vi "PlotGraph.vi"(0 "reference in":refnum<class "HTMLPlot.lvclass">, 5 "error in (no error)":errorcluster) -> (14 "reference out":refnum<class "HTMLPlot.lvclass">, 19 "error out":errorcluster)   [LabVIEW 2019, in "HTMLPlot.lvclass"]
uses:
  HTMLPlot.lvclass
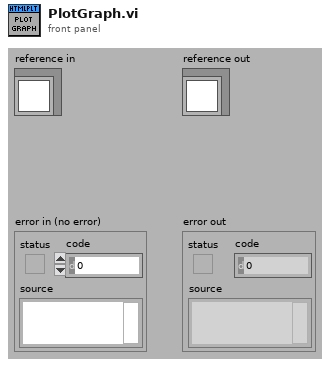
[diagram p1: front panel]
types:
  T1 = typedef "HTMLPlot.lvclass/ObjectAttributes.ctl" = cluster{"Attribute1":dbl, "GraphContainer":refnum<k7>, "ChartScriptFile":string, "UtilScriptFile(demoData)":string, "BaseHTML":string, "GenericProperties":cluster{"PlotType":T2, "PlotTitle":string, "XLabel":string, "YLabel":string, "ShowToolTip":bool}, "LegendProperties":cluster{"Show":bool, "Position":T3}, "BarPlot":cluster{"Dataset":dbl[][], "DatasetLabels":string[], "XLabels":string[], "PlotColours":u32[], "Stacked":bool}, "PiePlot":cluster{"Dataset":dbl[][], "DatasetLabels":string[], "PlotColours":u32[], "DoughnutStyle":bool, "PlotLabels":string[]}, "connection ID":refnum<k5>, "PortID":u64}
  T2 = typedef "HTMLPlot.lvclass/PlotType.ctl" = enum16{"bar", "line", "pie"}
  T3 = typedef "HTMLPlot.lvclass/LegendPosition.ctl" = enum16{"top", "right", "left", "bottom"}
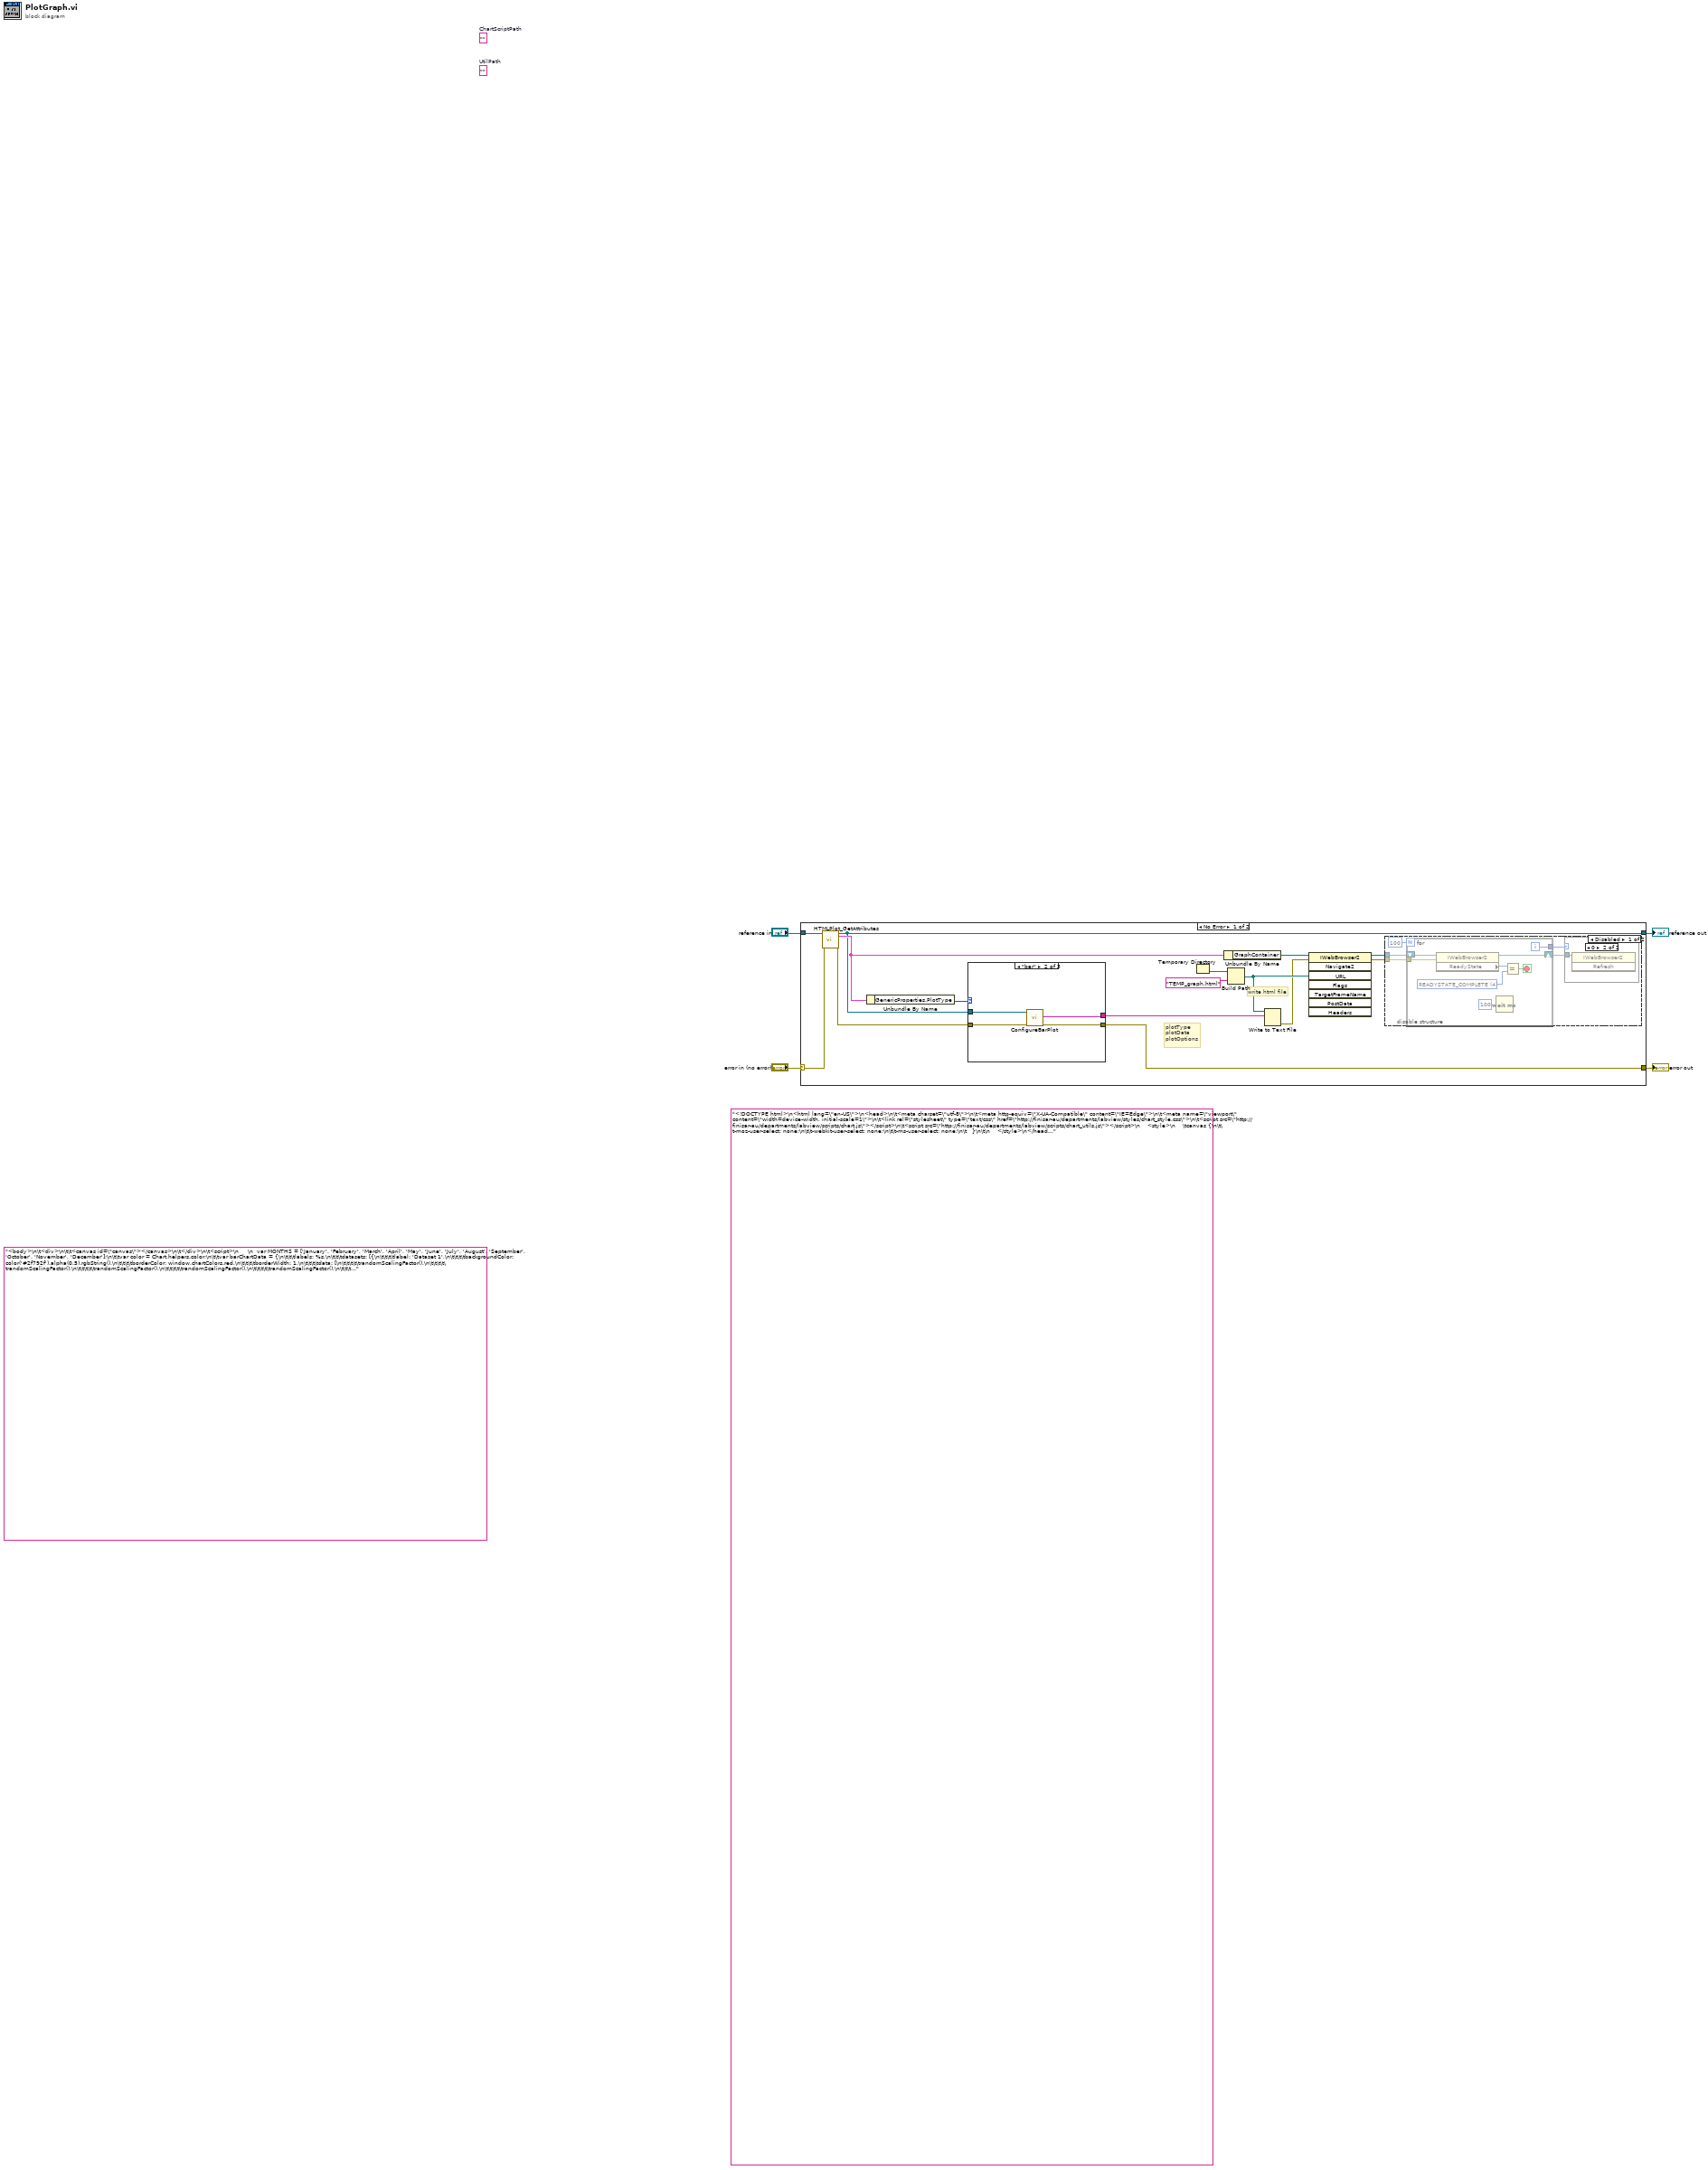
[diagram p0: block diagram]
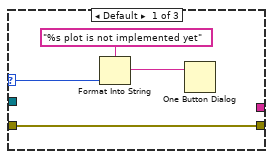
[diagram p2: hidden frame]
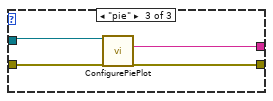
[diagram p3: hidden frame]
diagram:
  (unwired) ""  # UtilPath
  (unwired) ""  # ChartScriptPath
  (unwired) "<body>\n\t<div>\n\t\t<canvas id=\"canvas\"></canvas>\n\t</div>\n\t<script>\n     \n  var MONTHS = ['January', 'February', 'March', 'April', 'May', 'June', 'July', 'August', 'September', 'October', 'November', 'December'];\n\t\tvar color = Chart.helpers.color;\n\t\tvar barChartData = {\n\t\t\tlabels: %s,\n\t\t\tdatasets: [{\n\t\t\t\tlabel: 'Dataset 1',\n\t\t\t\tbackgroundColor: color('#2f792f').alpha(0.5).rgbString(),\n\t\t\t\tborderColor: window.chartColors.red,\n\t\t\t\tborderWidth: 1,\n\t\t\t\tdata: [\n\t\t\t\t\trandomScalingFactor(),\n\t\t\t\t\trandomScalingFactor(),\n\t\t\t\t\trandomScalingFactor(),\n\t\t\t\t\trandomScalingFactor(),\n\t\t\t\t\trandomScalingFactor(),\n\t\t\t\t\trandomScalingFactor(),\n\t\t\t\t\trandomScalingFactor()\n\t\t\t\t]\n\t\t\t}, {\n\t\t\t\tlabel: 'Dataset 2',\n\t\t\t\tbackgroundColor: color(window.chartColors.blue).alpha(0.5).rgbString(),\n\t\t\t\tborderColor: window.chartColors.blue,\n\t\t\t\tborderWidth: 1,\n\t\t\t\tdata: [\n\t\t\t\t\trandomScalingFactor(),\n\t\t\t\t\trandomScalingFactor(),\n\t\t\t\t\trandomScalingFactor(),\n\t\t\t\t\trandomScalingFactor(),\n\t\t\t\t\trandomScalingFactor(),\n\t\t\t\t\trandomScalingFactor(),\n\t\t\t\t\trandomScalingFactor()\n\t\t\t\t]\n\t\t\t}]\n\n\t\t};\n\n\t\twindow.onload = function() {\n\t\t\t//var ctx = document.getElementById('canvas').getContext('2d');\n\t\t\twindow.myBar = new Chart('canvas', {\n\t\t\t\ttype: 'bar',\n\t\t\t\tdata: barChartData,\n\t\t\t\toptions: {\n\t\t\t\t\tresponsive: true,\n\t\t\t\t\tlegend: {\n\t\t\t\t\t\tposition: 'top'\n\t\t\t\t\t},\n\t\t\t\t\ttitle: {\n\t\t\t\t\t\tdisplay: true,\n\t\t\t\t\t\ttext: 'Chart.js Bar Chart'\n\t\t\t\t\t},\n                    scales: {\n\t\t\t\t\t\txAxes: [{\n\t\t\t\t\t\t\tstacked: true,\n\t\t\t\t\t\t}],\n\t\t\t\t\t\tyAxes: [{\n\t\t\t\t\t\t\tstacked: true\n\t\t\t\t\t\t}]\n\t\t\t\t\t}\n\t\t\t\t}\n\t\t\t});\n\n\t\t};\n\n\n\t</script>\n</body>\n\n</html>\n\n\n"
  (unwired) "<!DOCTYPE html>\n<html lang=\"en-US\">\n<head>\n\t<meta charset=\"utf-8\">\n\t<meta http-equiv=\"X-UA-Compatible\" content=\"IE=Edge\">\n\t<meta name=\"viewport\" content=\"width=device-width, initial-scale=1\">\n\t<link rel=\"stylesheet\" type=\"text/css\" href=\"http://finisar-au/departments/labview/styles/chart_style.css\">\n\t<script src=\"http://finisar-au/departments/labview/scripts/chart.js\"></script>\n\t<script src=\"http://finisar-au/departments/labview/scripts/chart_utils.js\"></script>\n    <style>\n    \tcanvas {\n\t\t-moz-user-select: none;\n\t\t-webkit-user-select: none;\n\t\t-ms-user-select: none;\n\t   }\n\t\n    </style>\n</head>\n\n\n\n<body>\n\t<div id=\"container\" style=\"width: 75%;\">\n\t\t<canvas id=\"canvas\"></canvas>\n\t</div>\n\t<button id=\"randomizeData\">Randomize Data</button>\n\t<button id=\"addDataset\">Add Dataset</button>\n\t<button id=\"removeDataset\">Remove Dataset</button>\n\t<button id=\"addData\">Add Data</button>\n\t<button id=\"removeData\">Remove Data</button>\n\t<script>\n\t\tvar MONTHS = ['January', 'February', 'March', 'April', 'May', 'June', 'July', 'August', 'September', 'October', 'November', 'December'];\n\t\tvar color = Chart.helpers.color;\n        var Dataset1Color='#2f792f';\n\t\tvar barChartData = {\n\t\t\tlabels: ['January', 'February', 'March', 'April', 'May', 'June', 'July'],\n\t\t\tdatasets: [{\n\t\t\t\tlabel: 'Dataset 1',\n\t\t\t\tbackgroundColor: color('#2f792f').alpha(0.5).rgbString(),\n\t\t\t\tborderColor: window.chartColors.red,\n\t\t\t\tborderWidth: 1,\n\t\t\t\tdata: [\n\t\t\t\t\trandomScalingFactor(),\n\t\t\t\t\trandomScalingFactor(),\n\t\t\t\t\trandomScalingFactor(),\n\t\t\t\t\trandomScalingFactor(),\n\t\t\t\t\trandomScalingFactor(),\n\t\t\t\t\trandomScalingFactor(),\n\t\t\t\t\trandomScalingFactor()\n\t\t\t\t]\n\t\t\t}, {\n\t\t\t\tlabel: 'Dataset 2',\n\t\t\t\tbackgroundColor: color(window.chartColors.blue).alpha(0.5).rgbString(),\n\t\t\t\tborderColor: window.chartColors.blue,\n\t\t\t\tborderWidth: 1,\n\t\t\t\tdata: [\n\t\t\t\t\trandomScalingFactor(),\n\t\t\t\t\trandomScalingFactor(),\n\t\t\t\t\trandomScalingFactor(),\n\t\t\t\t\trandomScalingFactor(),\n\t\t\t\t\trandomScalingFactor(),\n\t\t\t\t\trandomScalingFactor(),\n\t\t\t\t\trandomScalingFactor()\n\t\t\t\t]\n\t\t\t}]\n\n\t\t};\n\n\t\twindow.onload = function() {\n\t\t\t//var ctx = document.getElementById('canvas').getContext('2d');\n\t\t\twindow.myBar = new Chart('canvas', {\n\t\t\t\ttype: 'bar',\n\t\t\t\tdata: barChartData,\n\t\t\t\toptions: {\n\t\t\t\t\tresponsive: true,\n\t\t\t\t\tlegend: {\n\t\t\t\t\t\tposition: 'top'\n\t\t\t\t\t},\n\t\t\t\t\ttitle: {\n\t\t\t\t\t\tdisplay: true,\n\t\t\t\t\t\ttext: 'Chart.js Bar Chart'\n\t\t\t\t\t},\n                    scales: {\n\t\t\t\t\t\txAxes: [{\n\t\t\t\t\t\t\tstacked: true,\n\t\t\t\t\t\t}],\n\t\t\t\t\t\tyAxes: [{\n\t\t\t\t\t\t\tstacked: true\n\t\t\t\t\t\t}]\n\t\t\t\t\t}\n\t\t\t\t}\n\t\t\t});\n\n\t\t};\n        \n\t\tdocument.getElementById('randomizeData').addEventListener('click', function() {\n\t\t\tvar zero = Math.random() < 0.2 ? true : false;\n\t\t\tbarChartData.datasets.forEach(function(dataset) {\n\t\t\t\tdataset.data = dataset.data.map(function() {\n\t\t\t\t\treturn zero ? 0.0 : randomScalingFactor();\n\t\t\t\t});\n\n\t\t\t});\n\t\t\twindow.myBar.update();\n\t\t});\n\n\t\tvar colorNames = Object.keys(window.chartColors);\n\t\tdocument.getElementById('addDataset').addEventListener('click', function() {\n\t\t\tvar colorName = colorNames[barChartData.datasets.length % colorNames.length];\n\t\t\tvar dsColor = window.chartColors[colorName];\n\t\t\tvar newDataset = {\n\t\t\t\tlabel: 'Dataset ' + (barChartData.datasets.length + 1),\n\t\t\t\tbackgroundColor: color(dsColor).alpha(0.5).rgbString(),\n\t\t\t\tborderColor: dsColor,\n\t\t\t\tborderWidth: 1,\n\t\t\t\tdata: []\n\t\t\t};\n\n\t\t\tfor (var index = 0; index < barChartData.labels.length; ++index) {\n\t\t\t\tnewDataset.data.push(randomScalingFactor());\n\t\t\t}\n\n\t\t\tbarChartData.datasets.push(newDataset);\n\t\t\twindow.myBar.update();\n\t\t});\n\n\t\tdocument.getElementById('addData').addEventListener('click', function() {\n\t\t\tif (barChartData.datasets.length > 0) {\n\t\t\t\tvar month = MONTHS[barChartData.labels.length % MONTHS.length];\n\t\t\t\tbarChartData.labels.push(month);\n\n\t\t\t\tfor (var index = 0; index < barChartData.datasets.length; ++index) {\n\t\t\t\t\t// window.myBar.addData(randomScalingFactor(), index);\n\t\t\t\t\tbarChartData.datasets[index].data.push(randomScalingFactor());\n\t\t\t\t}\n\n\t\t\t\twindow.myBar.update();\n\t\t\t}\n\t\t});\n\n\t\tdocument.getElementById('removeDataset').addEventListener('click', function() {\n\t\t\tbarChartData.datasets.pop();\n\t\t\twindow.myBar.update();\n\t\t});\n\n\t\tdocument.getElementById('removeData').addEventListener('click', function() {\n\t\t\tbarChartData.labels.splice(-1, 1); // remove the label first\n\n\t\t\tbarChartData.datasets.forEach(function(dataset) {\n\t\t\t\tdataset.data.pop();\n\t\t\t});\n\n\t\t\twindow.myBar.update();\n\t\t});\n\t</script>\n</body>\n\n</html>\n\n\n"
  n1 = case shown="No Error" "error in (no error)" {
    selector: "error in (no error)" -> [w19 w47]
    tunnel: [w6 w47] -> w3
    tunnel: [w9 w46] -> w1
    tunnel: "reference in" -> [w18 w46]
    frame No Error {
      # "plotType\nplotData\nplotOptions"
      # "write html file"
      n2 = call "HTMLPlot_GetAttributes.vi"("reference in"=w18, "error in (no error)"=w19) -> ("reference out"=w9:refnum<class "HTMLPlot.lvclass">, "Data"=w11:T1, "error out"=w7:errorcluster)  [unwired: 14 in, 1 out]
      n3 = Unbundle By Name(w11) -> ("GenericProperties.PlotType"=w10:T2)
      n4 = case shown="\"bar\"" w10 {
        selector: w10 -> [w23 _ _]
        tunnel: w9 -> [_ w26 w31]
        tunnel: [_ w27 w28] -> w8
        tunnel: w7 -> [w20 w25 w29]
        tunnel: [w20 w24 w30] -> w6
        frame Default {
          n5 = Format Into String(format string="%s plot is not implemented yet", w23) -> (resulting string=w21:string)  [unwired: 2 in, 1 out]
          n6 = One Button Dialog(message=w21) -> ()  [unwired: 1 in, 1 out]
        }
        frame "bar" {
          n7 = call "ConfigureBarPlot.vi"("reference in"=w26, "error in (no error)"=w25) -> ("fullHTML"=w27:string, "error out"=w24:errorcluster)  [unwired: 15 in, 1 out]
        }
        frame "pie" {
          n8 = call "ConfigurePiePlot.vi"("reference in"=w31, "error in (no error)"=w29) -> ("fullHTML"=w28:string, "error out"=w30:errorcluster)  [unwired: 15 in, 1 out]
        }
      }
      n9 = Temporary Directory() -> (w16:path)
      n10 = Unbundle By Name(w11) -> ("GraphContainer"=w17:refnum<k7>)
      n11 = Build Path(base path=w16, name or relative path="TEMP_graph.html") -> (appended path=w14:path)
      n12 = Write to Text File(file (use dialog)=w14, text=w8) -> (error out=w13:errorcluster)  [unwired: 2 in, 2 out]
      n13 = invoke class="IWebBrowser2" method="Navigate2"(reference=w17, error in=w13, "URL"=w14) -> (reference out=w12:refnum<k7>, error out=w5:errorcluster)  [unwired: 5 in, 6 out]
      n14 = disable-structure shown="Disabled" {
        disable-tunnel: w12 -> [w36 _]
        disable-tunnel: w5 -> [w32 _]
        frame Disabled {
          n15 = for {
            N: 100 -> [_]
            shift-right: [w44] -> w35
            shift-left: w36 -> [w45]
            tunnel: [w39] -> w33
            tunnel: w32 -> [w38]
            i -> [w39]
            stop <- w40 stop-if-true
            w42 = 4 items=["READYSTATE_UNINITIALIZED", "READYSTATE_LOADING", "READYSTATE_LOADED", "READYSTATE_INTERACTIVE", "READYSTATE_COMPLETE"] ("ReadyState")
            n16 = property class="IWebBrowser2"(reference=w45, error in=w38) -> (reference out=w44:refnum<k7>, "ReadyState"=w43:i32)  [unwired: 1 out]
            n17 = Wait (ms)(milliseconds to wait=u32 100) -> ()  [unwired: 1 out]
            n18 = Equal?(x=w43, y=w42) -> (x = y?=w40:bool)
          }
          n19 = case shown="0" w33 {
            tunnel: w35 -> [_ w37]
            frame Default {
            }
            frame 0 {
              n20 = invoke class="IWebBrowser2" method="Refresh"(reference=w37) -> ()  [unwired: 2 in, 3 out]
            }
          }
        }
        frame Enabled {
        }
      }
    }
    frame Error {
    }
  }
  "error out" <- w3
  "reference out" <- w1
